vi "Close Project.vi"(8 "error in (no error)":errorcluster, 10 "Project Path in":path, 11 "Application reference":refnum<vi>) -> (0 "error out":errorcluster, 2 "Project Path out":path, 3 "Application out":refnum<vi>)   [LabVIEW 2019, in "gRPC Scripting Tools.lvlib"]
uses:
  gRPC Scripting Tools.lvlib
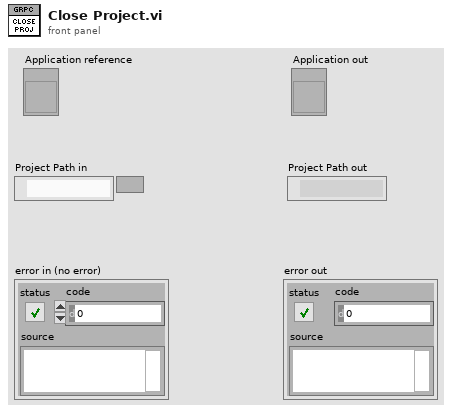
[diagram p1: front panel]
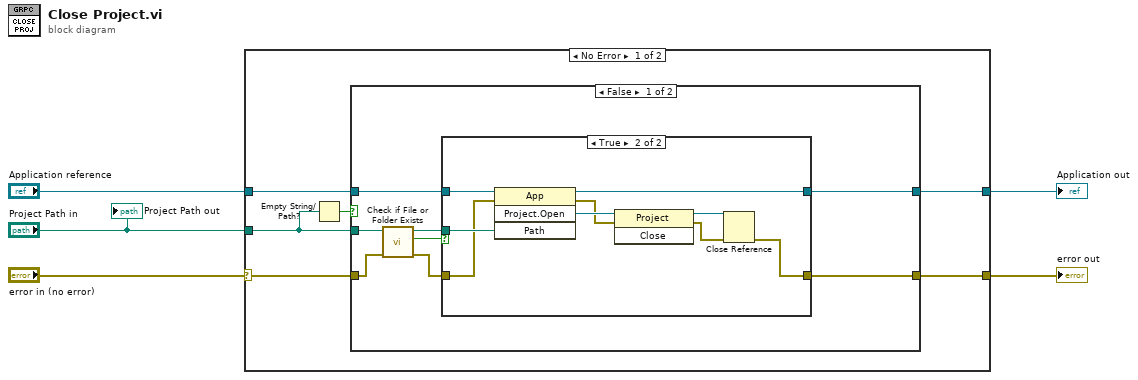
[diagram p0: block diagram]
diagram:
  n1 = case shown="No Error" "error in (no error)" {
    selector: "error in (no error)" -> [w10 w33]
    tunnel: "Project Path in" -> [w8 _]
    tunnel: [w9 _] -> w4
    tunnel: [w11 w33] -> w3
    tunnel: "Application reference" -> [w6 _]
    frame No Error {
      n2 = Empty String/Path?(string/path=w8) -> (empty?=w7:bool)
      n3 = case shown="False" w7 {
        tunnel: w8 -> [w19 _]
        tunnel: [w16 w31] -> w11
        tunnel: w10 -> [w15 w31]
        tunnel: [w14 w32] -> w9
        tunnel: w6 -> [w13 w32]
        frame False {
          n4 = call <vilib>:"Check if File or Folder Exists.vi"("error in (no error)"=w15, "path"=w19) -> ("error out"=w17:errorcluster, "file or folder exists?"=w12:bool, "dup path"=w18:path)  [unwired: 7 in]
          n5 = case shown="True" w12 {
            tunnel: w18 -> [_ w30]
            tunnel: w17 -> [w20 w29]
            tunnel: [w20 w22] -> w16
            tunnel: [w21 w26] -> w14
            tunnel: w13 -> [w21 w25]
            frame False {
            }
            frame True {
              n6 = invoke class="App" method="Project.Open"(reference=w25, error in=w29, "Path"=w30) -> (reference out=w26:refnum<vi>, error out=w27:errorcluster, "Project:Open"=w28:refnum<vi>)  [unwired: 1 in, 1 out]
              n7 = invoke class="Project" method="Close"(reference=w28, error in=w27) -> (reference out=w23:refnum<vi>, error out=w24:errorcluster)  [unwired: 1 in, 1 out]
              n8 = Close Reference(reference=w23, error in (no error)=w24) -> (error out=w22:errorcluster)
            }
          }
        }
        frame True {
        }
      }
    }
    frame Error {
    }
  }
  "error out" <- w3
  "Application out" <- w4
  "Project Path out" <- "Project Path in"
